vi "Main.vi"() -> ()   [LabVIEW 2015]
uses:
  Game States.ctl
  Game Data.ctl
  <vilib>/MakerHub/LINX/Private/Type Defs/User Platform.ctl
  <vilib>/MakerHub/LINX/Private/Type Defs/Interface.ctl
  <vilib>/Utility/miscctls.llb/LV3DPointTypeDef.ctl
  3D Point.ctl
  Level/Level.lvclass/Level.ctl
  <vilib>/MakerHub/LINX/Public/Peripherals/Analog/Analog Read 1 Chan.vi
  Player/Player.lvclass
  Level/Level.lvclass
  3D Object/3D Object.lvclass
  Input/Input.lvclass
  3D Scene/3D Scene.lvclass
  Render Window/Render Window.lvclass
  Control Window/Control Window.lvclass
  <vilib>/MakerHub/LINX/LMH-LINX.lvlib
panel:
  out "Step?":bool
  in  "Use Hardware":bool
  out "Error Out":errorcluster
  in  "Error In":errorcluster
  in  "Serial Port":refnum<visa-resource-name>="COM4"
  out "Yaw":sgl
  out "Pitch":sgl
  out "error out":errorcluster
  in  "Display":enum16{"Control Window", "Render Window"}(ring)
  out "3D Debug":refnum<vi>(3d-picture)
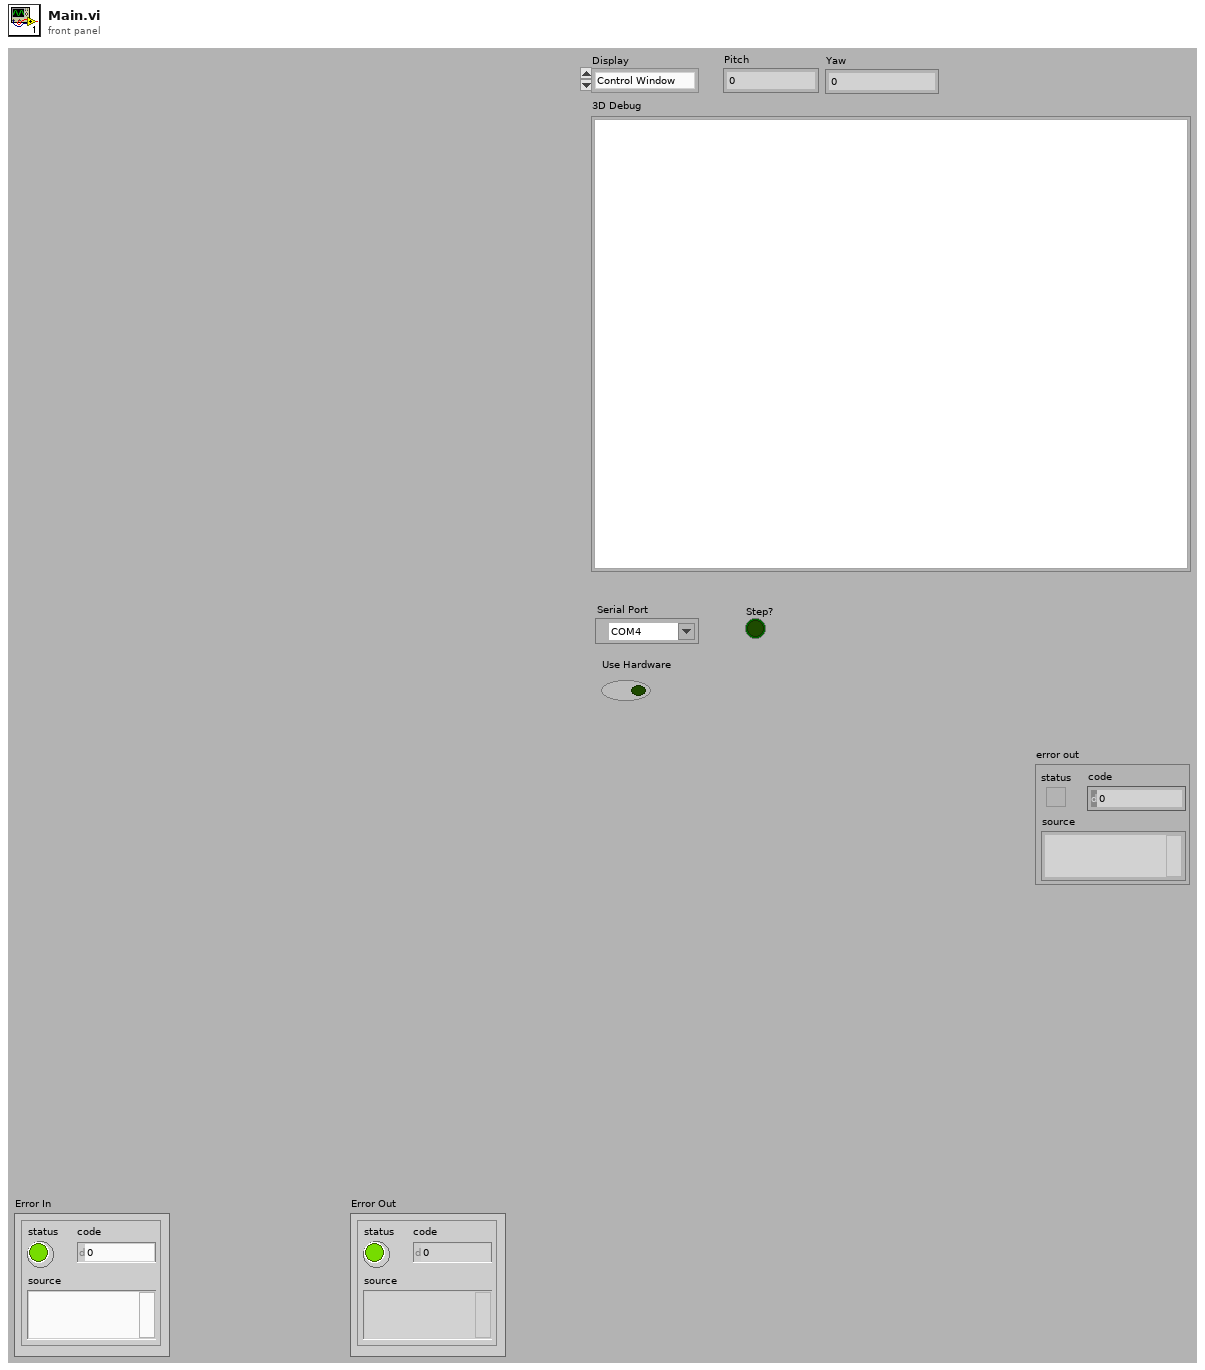
[diagram p1: front panel]
types:
  T1 = typedef "Game Data.ctl" = cluster{"Current Tick Count":u32, "Ticks From Start":u32}
  T2 = typedef "Game States.ctl" = enum16{"Initialize", "Get Input", "Draw Scene", "Shutdown"}
  T3 = typedef "LMH-LINX.lvlib/Interface.ctl" = enum16{"Serial", "TCP"}
  T4 = typedef "LMH-LINX.lvlib/User Platform.ctl" = enum16{"Default", "LINX", "myRIO"}
  T5 = typedef "LMH-LINX.lvlib/LINX Ref.ctl" = cluster{"Platform":T6, "Interface":T3, "LINX Device Config":T7}
  T6 = typedef "LMH-LINX.lvlib/Platform.ctl" = enum16{"LINX", "myRIO"}
  T7 = typedef "LMH-LINX.lvlib/Device.lvlib/LINX Device Config.ctl" = cluster{"Interface":T3, "COM Port":refnum<visa-resource-name>, "TCP Configuration":T8, "Device Family":u8, "Device ID":u8, "Device Name":string, "TCP Ref":refnum<k5>, "Channels":T9}
  T8 = typedef "LMH-LINX.lvlib/Device.lvlib/TCP Config.ctl" = cluster{"IP Address":string, "Port":u16}
  T9 = typedef "LMH-LINX.lvlib/Channels.ctl" = cluster{"DI":u8[], "DO":u8[], "AI":u8[], "AO":u8[], "PWM":u8[], "QE":u8[], "UART":u8[], "I2C 2":u8[], "SPI":u8[], "CAN":u8[], "Servo":u8[], "AI Ref (V)":dbl, "AO Ref (V)":dbl, "AO Resolution (Bits)":u8}
  T10 = typedef "3D Point.ctl" = cluster{"X":sgl, "Y":sgl, "Z":sgl}
  T11 = typedef "LV3DPointTypeDef.ctl" = cluster{"X":sgl, "Y":sgl, "Z":sgl}
  T12 = enum16{"None", "Spherical", "Flying", "Oriented"}
  T13 = enum16{"Open", "Minimized", "Maximized", "Hidden"}
  T14 = typedef "Level.lvclass/Segment.ctl" = cluster{"Point 1":T15, "Point 2":T15}
  T15 = typedef "Level.lvclass/Point.ctl" = cluster{"Z":dbl, "X":dbl}
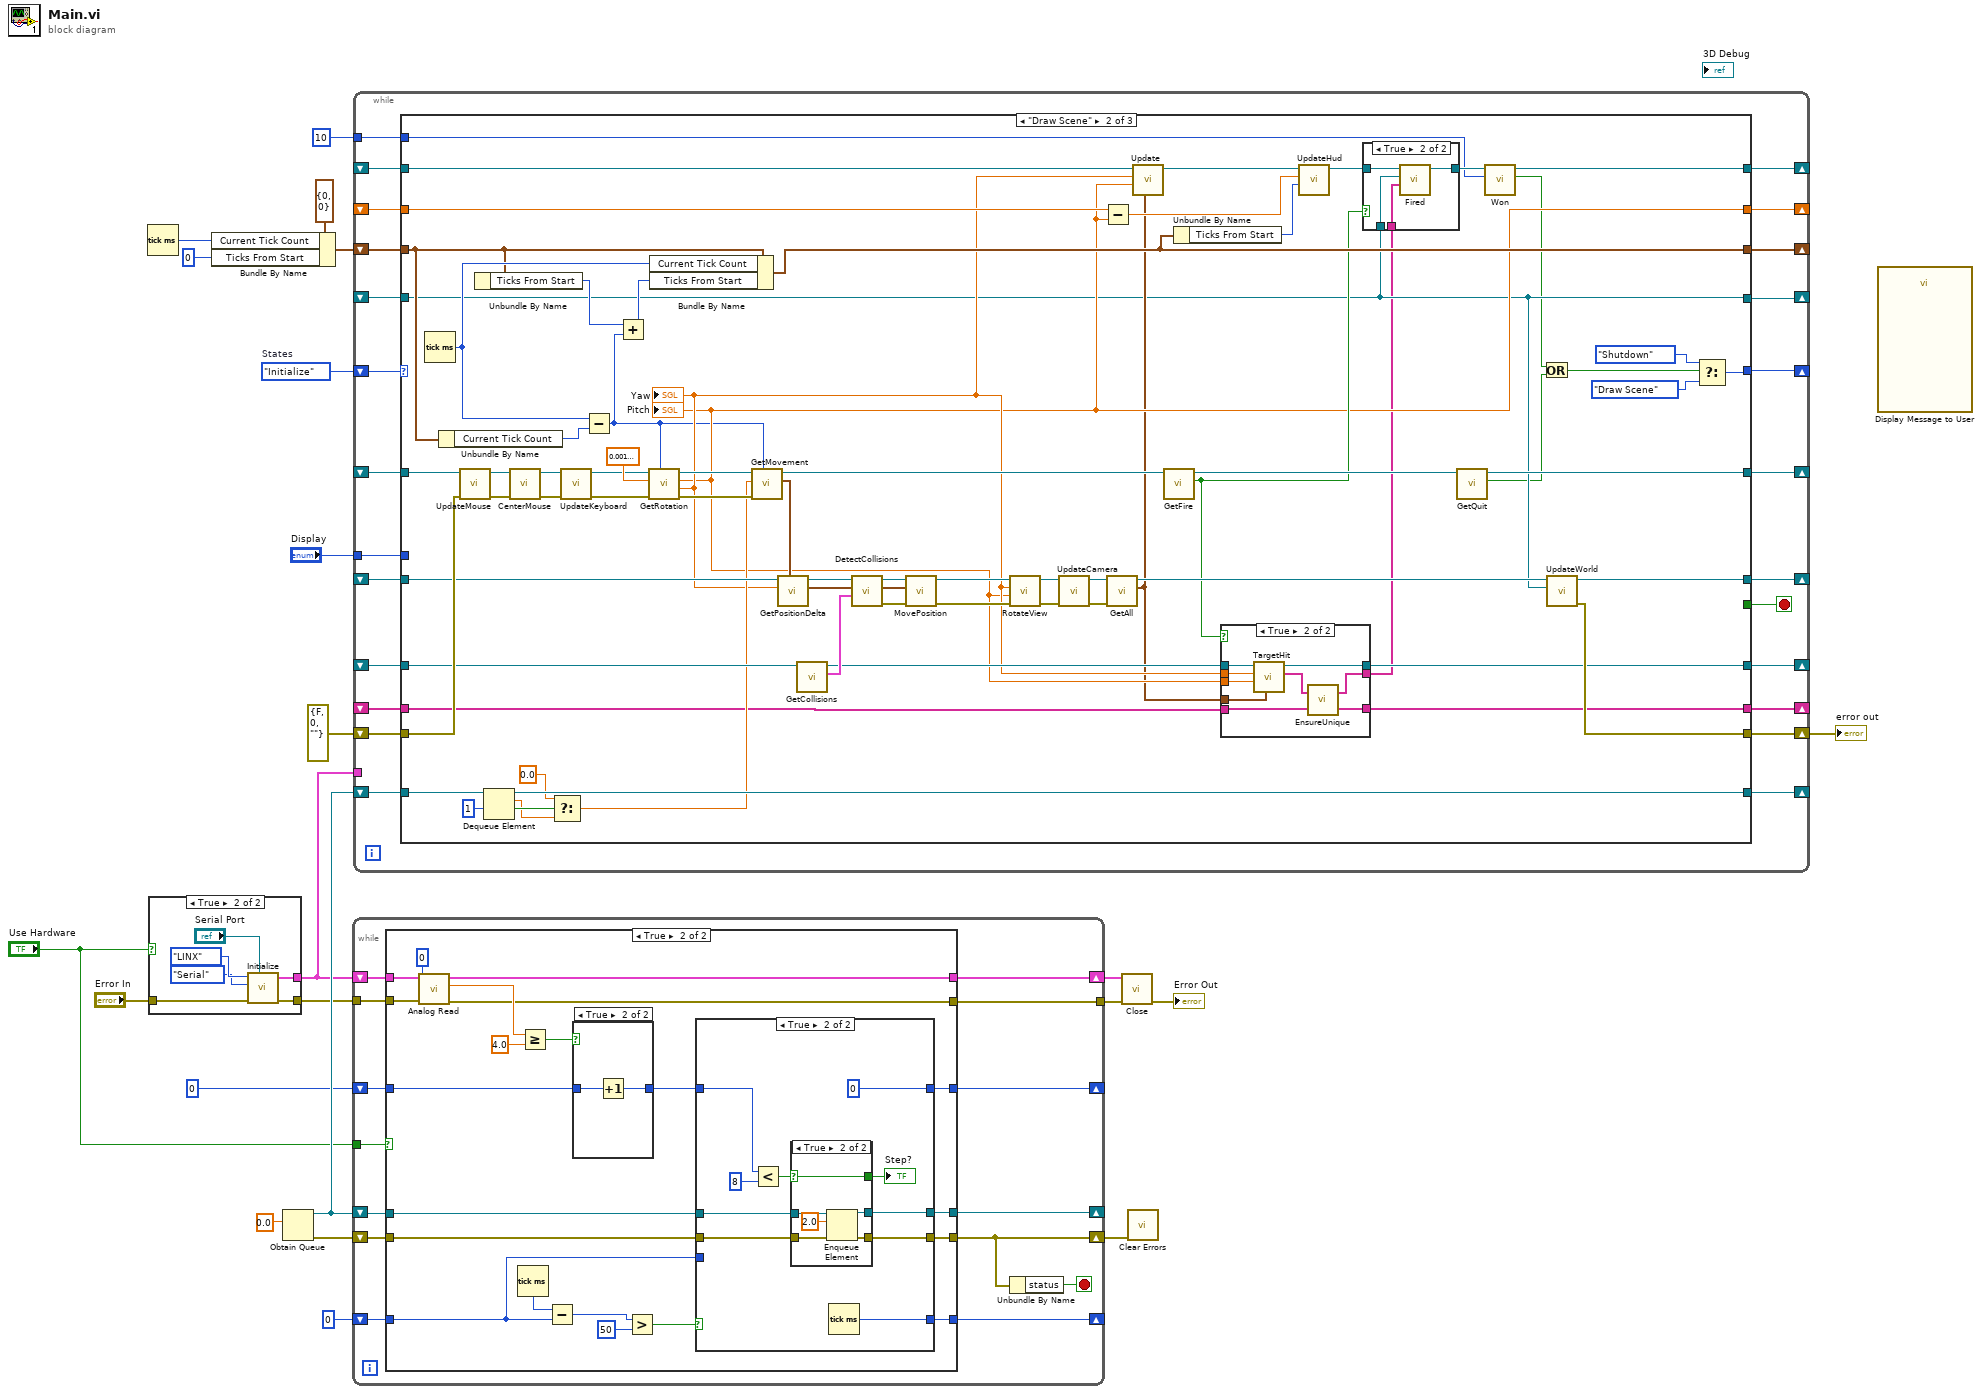
[diagram p0: block diagram]
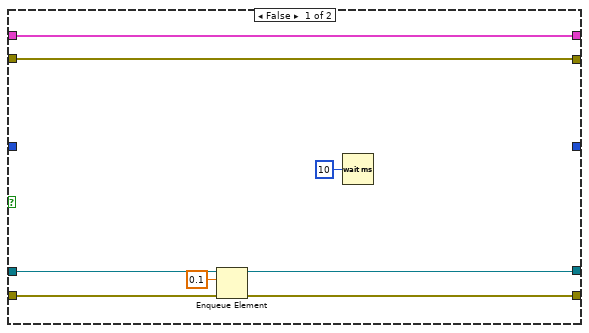
[diagram p3: hidden frame]
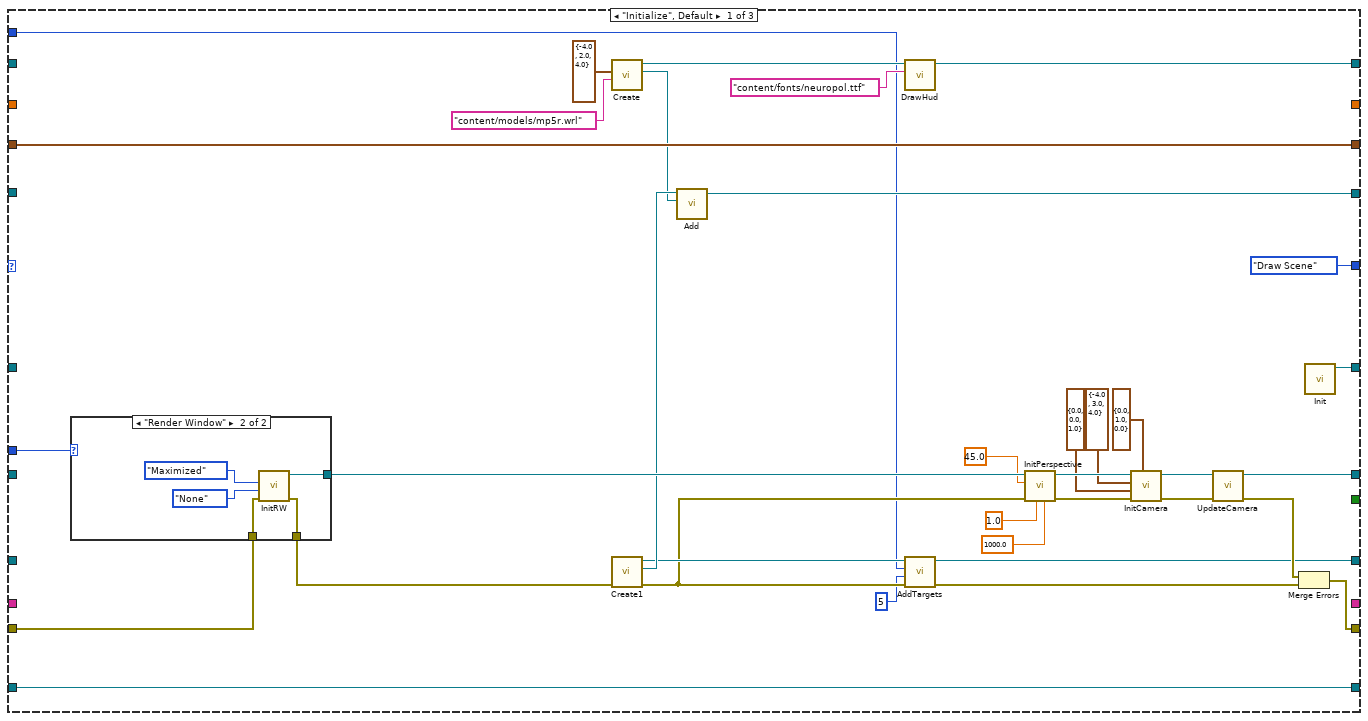
[diagram p7: hidden frame]
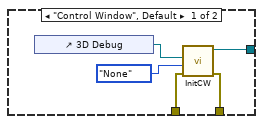
[diagram p8: hidden frame]
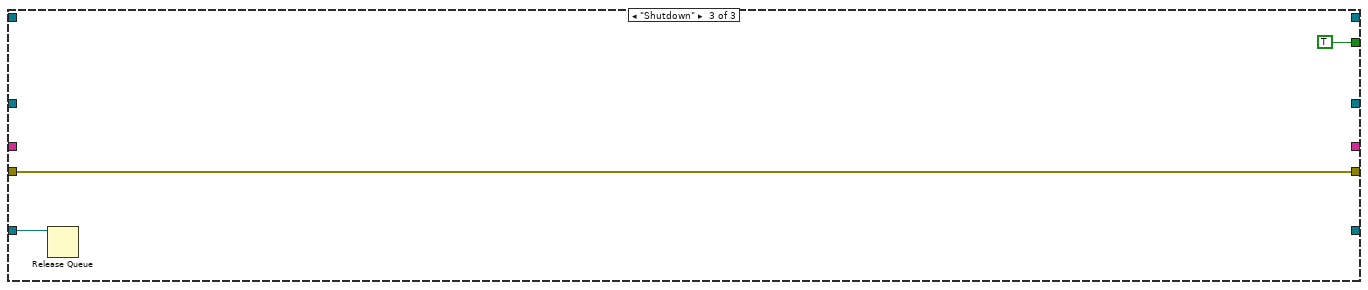
[diagram p11: hidden frame]
diagram:
  w22 = Game_States."Initialize"  # States
  n1 = Tick Count (ms)() -> (millisecond timer value=w3:u32)
  n2 = case shown="True" "Use Hardware" {
    tunnel: [_ w29] -> w15
    tunnel: [w23 w26] -> w11
    tunnel: "Error In" -> [w23 w24]
    frame False {
    }
    frame True {
      n3 = call <vilib>:"Initialize.vi"("Serial Port"="Serial Port", "Error In"=w24, "Interface"=Interface."Serial", "Platform"=User_Platform."LINX") -> ("Error Out"=w26:errorcluster, "LINX Ref"=w29:T5)  [unwired: 5 in, 1 out]
    }
  }
  n4 = Bundle By Name(cluster=T1 {"Current Tick Count"=0, "Ticks From Start"=0} ("Data"), "Current Tick Count"=w3, "Ticks From Start"=u32 0) -> (w18:T1)
  n5 = Obtain Queue(element data type=0.0) -> (queue out=w16:refnum<queue>, error out=w8:errorcluster)  [unwired: 4 in, 1 out]
  n6 = while {
    shift-right: [w42] -> w14
    shift-left: w15 -> [w43]
    shift-right: [w40] -> _
    shift-left: 0 -> [w41]
    shift-right: [w38] -> _
    shift-left: 0 -> [w39]
    tunnel: w11 -> [w37]
    tunnel: [w36] -> w10
    shift-right: [w32] -> w7
    shift-left: w8 -> [w33]
    shift-right: [w34] -> _
    shift-left: w16 -> [w35]
    tunnel: "Use Hardware" -> [w30]
    stop <- w31 stop-if-true
    n7 = case shown="True" w30 {
      tunnel: w43 -> [w51 w72]
      tunnel: [w51 w71] -> w42
      tunnel: w41 -> [_ w66]
      tunnel: [_ w60] -> w40
      tunnel: w39 -> [_ w59]
      tunnel: [_ w58] -> w38
      tunnel: w37 -> [w50 w57]
      tunnel: [w50 w56] -> w36
      tunnel: w35 -> [w49 w55]
      tunnel: [w48 w54] -> w34
      tunnel: w33 -> [w47 w53]
      tunnel: [w46 w52] -> w32
      frame False {
        n8 = Enqueue Element(queue=w49, element=0.1, error in (no error)=w47) -> (queue out=w48:refnum<queue>, error out=w46:errorcluster)  [unwired: 1 in, 1 out]
        n9 = Wait (ms)(milliseconds to wait=u32 10) -> ()  [unwired: 1 out]
      }
      frame True {
        n10 = call-poly <vilib>:"Analog Read.vi"("Error In"=w57, "Analog Channel"=u8 0, "LINX Resource"=w72) -> ("Error Out"=w56:errorcluster, "AI Value"=w69:dbl, "LINX Resource"=w71:T5)  [unwired: 5 in, 1 out]
        n11 = Tick Count (ms)() -> (millisecond timer value=w65:u32)
        n12 = Greater Or Equal?(x=w69, y=4.0) -> (x >= y?=w67:bool)
        n13 = Subtract(x=w65, y=w59) -> (x-y=w64:u32)
        n14 = case shown="True" w67 {
          tunnel: w66 -> [w95 w97]
          tunnel: [w95 w96] -> w61
          frame False {
          }
          frame True {
            n15 = Increment(x=w97) -> (x+1=w96:i32)
          }
        }
        n16 = Greater?(x=w64, y=u32 50) -> (0:w62:bool)
        n17 = case shown="True" w62 {
          tunnel: w61 -> [w76 w84]
          tunnel: [w76 0] -> w60
          tunnel: w59 -> [w75 _]
          tunnel: [w75 w85] -> w58
          tunnel: w55 -> [w74 w82]
          tunnel: [w74 w81] -> w54
          tunnel: w53 -> [w73 w80]
          tunnel: [w73 w79] -> w52
          frame False {
          }
          frame True {
            n18 = Less?(x=w84, y=8) -> (x < y?=w78:bool)
            n19 = case shown="True" w78 {
              selector: w78 -> [_ w89]
              tunnel: w82 -> [w88 w94]
              tunnel: [w88 w93] -> w81
              tunnel: w80 -> [w87 w92]
              tunnel: [w87 w91] -> w79
              tunnel: [_ w89] -> w77
              frame False {
              }
              frame True {
                n20 = Enqueue Element(queue=w94, element=2.0, error in (no error)=w92) -> (queue out=w93:refnum<queue>, error out=w91:errorcluster)  [unwired: 1 in, 1 out]
              }
            }
            "Step?" <- w77
            n21 = Tick Count (ms)() -> (millisecond timer value=w85:u32)
          }
        }
      }
    }
    n22 = Unbundle By Name(w32) -> ("status"=w31:bool)
  }
  n23 = while {
    shift-right: [w121] -> _
    shift-left: w22 -> [w122]
    tunnel: "Display" -> [w119]
    shift-right: [w118] -> _
    shift-left: _ -> [w117]
    shift-right: [w115] -> _
    shift-left: _ -> [w114]
    shift-right: [w112] -> _
    shift-left: w18 -> [w113]
    shift-right: [w111] -> _
    shift-left: _ -> [w110]
    shift-right: [w107] -> _
    shift-left: _ -> [w108]
    shift-right: [w109] -> w17
    shift-left: errorcluster {"status"=FALSE, "code"=0, "source"=""} ("error in (no error)") -> [w116]
    shift-right: [w105] -> _
    shift-left: w16 -> [w106]
    tunnel: w15 -> [_]
    shift-right: [w104] -> _
    shift-left: _ -> [w103]
    shift-right: [w102] -> _
    shift-left: _ -> [w101]
    tunnel: 10 ("Num Targets") -> [w100]
    shift-right: [w98] -> _
    shift-left: _ -> [w99]
    stop <- w120 stop-if-true
    n24 = case shown="\"Draw Scene\"" w122 {
      tunnel: [Game_States."Draw Scene" ("States") w232 _] -> w121
      tunnel: [_ _ TRUE] -> w120
      tunnel: w119 -> [w156 _ _]
      tunnel: [w147 w230 _] -> w118
      tunnel: w117 -> [_ w205 _]
      tunnel: w116 -> [w140 w218 w256]
      tunnel: [w149 w234 _] -> w115
      tunnel: w114 -> [_ w229 _]
      tunnel: w113 -> [w152 w191 _]
      tunnel: [w152 w192 _] -> w112
      tunnel: [w145 w178 _] -> w111
      tunnel: w110 -> [_ w178 _]
      tunnel: [w136 w227 w256] -> w109
      tunnel: w108 -> [_ w209 _]
      tunnel: [w125 w183 _] -> w107
      tunnel: w106 -> [w141 w204 w255]
      tunnel: [w141 w202 _] -> w105
      tunnel: [w130 w176 _] -> w104
      tunnel: w103 -> [_ w197 _]
      tunnel: [_ w180 _] -> w102
      tunnel: w101 -> [_ w195 _]
      tunnel: w100 -> [w123 w175 _]
      tunnel: w99 -> [_ w170 _]
      tunnel: [_ w169 _] -> w98
      frame "Initialize", Default {
        n25 = case shown="\"Render Window\"" w156 {
          tunnel: [w160 w165] -> w155
          tunnel: w140 -> [w159 w164]
          tunnel: [w158 w163] -> w139
          frame "Control Window", Default {
            n26 = control-ref of="3D Debug"() -> (w161:refnum<vi>)
            n27 = call "InitCW.vi"("error in (no error)"=w159, "Camera Controller"=T12."None", "SceneGraphDisp"=w161) -> ("error out"=w158:errorcluster, "Control Window out"=w160:refnum<class "Control Window.lvclass">)  [unwired: 7 in]
          }
          frame "Render Window" {
            n28 = call "InitRW.vi"("error in (no error)"=w164, "Camera Controller"=enum16{"None", "Spherical", "Flying"}."None", "Window State"=T13."Maximized") -> ("error out"=w163:errorcluster, "Render Window out"=w165:refnum<class "Render Window.lvclass">)  [unwired: 7 in]
          }
        }
        n29 = call "Create.vi"("Gun VRML"="content/models/mp5r.wrl", "Position"=T10 {"X"=-4.0, "Y"=2.0, "Z"=4.0}) -> ("Model"=w132:refnum<class "3D Object.lvclass">, "Player out"=w131:refnum<class "Player.lvclass">)  [unwired: 7 in, 1 out]
        n30 = call "Create1.vi"("error in (no error)"=w139) -> ("error out"=w127:errorcluster, "Model"=w133:refnum<class "3D Object.lvclass">, "Level out"=w128:refnum<class "Level.lvclass">)  [unwired: 8 in]
        n31 = call "Add.vi"("Child in"=w132, "Parent in"=w133) -> ("Parent out"=w145:refnum<class "3D Object.lvclass">)  [unwired: 7 in, 2 out]
        n32 = call "DrawHud.vi"("Font"="content/fonts/neuropol.ttf", "Player in"=w131) -> ("Player out"=w130:refnum<class "Player.lvclass">)  [unwired: 8 in, 1 out]
        n33 = call "AddTargets.vi"("error in (no error)"=w127, "Difficulty"=u8 5, "Num Targets"=w123, "Level in"=w128) -> ("error out"=w126:errorcluster, "Level out"=w125:refnum<class "Level.lvclass">)  [unwired: 6 in]
        n34 = call-dynamic "InitPerspective.vi"("Far Clipping"=sgl 1000.0, "Near Clipping"=sgl 1.0, "error in (no error)"=w127, "FOV"=sgl 45.0, "3D Scene in"=w155) -> ("error out"=w143:errorcluster, "3D Scene out"=w151:refnum<class "3D Scene.lvclass">)  [unwired: 5 in]
        n35 = call "InitCamera.vi"("Up Direction"=T11 {"X"=0.0, "Y"=1.0, "Z"=0.0}, "error in (no error)"=w143, "Target"=T11 {"X"=0.0, "Y"=0.0, "Z"=1.0}, "Camera Position"=T11 {"X"=-4.0, "Y"=3.0, "Z"=4.0}, "3D Scene in"=w151) -> ("error out"=w144:errorcluster, "3D Scene out"=w148:refnum<class "3D Scene.lvclass">)  [unwired: 5 in]
        n36 = call-dynamic "UpdateCamera.vi"("error in (no error)"=w144, "3D Scene in"=w148) -> ("error out"=w137:errorcluster, "3D Scene out"=w147:refnum<class "3D Scene.lvclass">)  [unwired: 8 in]
        n37 = Merge Errors(w137, w126) -> (w136:errorcluster)
        n38 = call "Init.vi"() -> ("Input out"=w149:refnum<class "Input.lvclass">)  [unwired: 10 in, 1 out]
      }
      frame "Draw Scene" {
        n39 = Tick Count (ms)() -> (millisecond timer value=w235:u32)
        n40 = Unbundle By Name(w191) -> ("Current Tick Count"=w236:u32)
        n41 = call "UpdateMouse.vi"("error in (no error)"=w218, "Input in"=w229) -> ("error out"=w225:errorcluster, "Input out"=w226:refnum<class "Input.lvclass">)  [unwired: 8 in]
        n42 = Unbundle By Name(w191) -> ("Ticks From Start"=w190:u32)
        n43 = Dequeue Element(queue=w204, timeout in ms (-1)=1) -> (queue out=w202:refnum<queue>, element=w200:dbl, timed out?=w201:bool)  [unwired: 1 in, 1 out]
        n44 = call "CenterMouse.vi"("error in (no error)"=w225, "Input in"=w226) -> ("error out"=w221:errorcluster, "Input out"=w224:refnum<class "Input.lvclass">)  [unwired: 8 in]
        n45 = Select(t=0.0, s=w201, f=w200) -> (s? t:f=w199:dbl)
        n46 = call "UpdateKeyboard.vi"("error in (no error)"=w221, "Input in"=w224) -> ("error out"=w222:errorcluster, "Input out"=w223:refnum<class "Input.lvclass">)  [unwired: 8 in]
        n47 = Subtract(x=w235, y=w236) -> (x-y=w168:u32)
        n48 = Add(x=w190, y=w168) -> (x+y=w189:u32)
        n49 = call "GetRotation.vi"("Game Ticks"=w168, "error in (no error)"=w222, "Rotation Speed"=sgl 0.001, "Input in"=w223) -> ("error out"=w228:errorcluster, "Yaw"=w181:sgl, "Pitch"=w180:sgl, "Input out"=w237:refnum<class "Input.lvclass">)  [unwired: 4 in]
        "Pitch" <- w180
        "Yaw" <- w181
        n50 = Bundle By Name(cluster=w191, "Current Tick Count"=w235, "Ticks From Start"=w189) -> (w192:T1)
        n51 = call "GetMovement.vi"("Game Ticks"=w168, "error in (no error)"=w228, "Move Speed"=w199, "Input in"=w237) -> ("Move Vector"=w213:cluster{"[0]":sgl, "[1]":sgl, "[2]":sgl}, "Input out"=w188:refnum<class "Input.lvclass">)  [unwired: 5 in, 1 out]
        n52 = call "GetPositionDelta.vi"("Move Vector"=w213, "Yaw"=w181, "3D Scene in"=w205) -> ("Position Delta"=w207:cluster{"X":sgl, "Y":sgl, "Z":sgl}, "3D Scene out"=w212:refnum<class "3D Scene.lvclass">)  [unwired: 6 in, 1 out]
        n53 = call "GetCollisions.vi"("Level in"=w209) -> ("Collisions"=w208:T14[], "Level out"=w184:refnum<class "Level.lvclass">)  [unwired: 8 in, 1 out]
        n54 = call "DetectCollisions.vi"("Collision Points"=w208, "Position Delta"=w207, "3D Scene in"=w212) -> ("error out"=w210:errorcluster, "Adjusted Position Delta"=w206:cluster{"X":sgl, "Y":sgl, "Z":sgl}, "3D Scene out"=w211:refnum<class "3D Scene.lvclass">)  [unwired: 6 in]
        n55 = call "MovePosition.vi"("error in (no error)"=w210, "Position Delta"=w206, "3D Scene in"=w211) -> ("error out"=w216:errorcluster, "3D Scene out"=w217:refnum<class "3D Scene.lvclass">)  [unwired: 7 in]
        n56 = call "RotateView.vi"("error in (no error)"=w216, "Pitch"=w180, "Yaw"=w181, "3D Scene in"=w217) -> ("error out"=w214:errorcluster, "3D Scene out"=w215:refnum<class "3D Scene.lvclass">)  [unwired: 6 in]
        n57 = call-dynamic "UpdateCamera.vi"("error in (no error)"=w214, "3D Scene in"=w215) -> ("error out"=w219:errorcluster, "3D Scene out"=w220:refnum<class "3D Scene.lvclass">)  [unwired: 8 in]
        n58 = Subtract(x=w195, y=w180) -> (x-y=w194:sgl)
        n59 = call "GetAll.vi"("error in (no error)"=w219, "3D Scene in"=w220) -> ("Position"=w179:T10, "3D Scene out"=w185:refnum<class "3D Scene.lvclass">)  [unwired: 5 in, 3 out]
        n60 = call "Update.vi"("New Position"=w179, "Pitch"=w180, "Yaw"=w181, "Player in"=w197) -> ("Player out"=w196:refnum<class "Player.lvclass">)  [unwired: 6 in, 1 out]
        n61 = call "GetFire.vi"("Input in"=w188) -> ("Fire?"=w182:bool, "Input out"=w187:refnum<class "Input.lvclass">)  [unwired: 8 in, 1 out]
        n62 = Unbundle By Name(w192) -> ("Ticks From Start"=w193:u32)
        n63 = case shown="True" w182 {
          tunnel: w184 -> [w240 w249]
          tunnel: [w240 w248] -> w183
          tunnel: w181 -> [_ w247]
          tunnel: w180 -> [_ w246]
          tunnel: w179 -> [_ w245]
          tunnel: [_ w243] -> w171
          tunnel: w170 -> [w239 w241]
          tunnel: [w239 w242] -> w169
          frame False {
          }
          frame True {
            n64 = call "TargetHit.vi"("Position"=w245, "Pitch"=w246, "Yaw"=w247, "Level in"=w249) -> ("Hit Targets"=w244:string[], "Level out"=w248:refnum<class "Level.lvclass">)  [unwired: 5 in, 1 out]
            n65 = call "EnsureUnique.vi"("Existing Targets Hit"=w241, "Potentially New Targets Hit"=w244) -> ("Existing Targets Hit Updated"=w242:string[], "New Targets Hit"=w243:string[])
          }
        }
        n66 = call "UpdateHud.vi"("Ticks Elapsed (ms)"=w193, "Pitch Delta"=w194, "Player in"=w196) -> ("Player out"=w186:refnum<class "Player.lvclass">)  [unwired: 7 in, 1 out]
        n67 = case shown="True" w182 {
          tunnel: w186 -> [w250 w254]
          tunnel: [w250 w253] -> w177
          tunnel: w171 -> [_ w252]
          tunnel: w178 -> [_ w251]
          frame False {
          }
          frame True {
            n68 = call "Fired.vi"("Hit Targets"=w252, "World In"=w251, "Player in"=w254) -> ("Player out"=w253:refnum<class "Player.lvclass">)  [unwired: 7 in, 1 out]
          }
        }
        n69 = call "GetQuit.vi"("Input in"=w187) -> ("Quit?"=w174:bool, "Input out"=w234:refnum<class "Input.lvclass">)  [unwired: 8 in, 1 out]
        n70 = call "Won.vi"("Num Targets"=w175, "Player in"=w177) -> ("Won?"=w173:bool, "Player out"=w176:refnum<class "Player.lvclass">)  [unwired: 7 in, 1 out]
        n71 = Or(x=w173, y=w174) -> (x .or. y?=w172:bool)
        n72 = call-dynamic "UpdateWorld.vi"("World in"=w178, "3D Scene in"=w185) -> ("error out"=w227:errorcluster, "3D Scene out"=w230:refnum<class "3D Scene.lvclass">)  [unwired: 8 in]
        n73 = Select(t=Game_States."Shutdown" ("States"), s=w172, f=Game_States."Draw Scene") -> (s? t:f=w232:T2)
      }
      frame "Shutdown" {
        n74 = Release Queue(queue=w255) -> ()  [unwired: 2 in, 3 out]
      }
    }
  }
  "error out" <- w17
  n75 = call <vilib>:"Close.vi"("Error In"=w10, "LINX Resource"=w14) -> ("Error Out"=→"Error Out":errorcluster)  [unwired: 8 in, 1 out]
  n76 = call <vilib>:"Clear Errors.vi"("error in (no error)"=w7) -> ()  [unwired: 5 in, 2 out]
  n77 = call "Display Message to User"() -> ()  [unwired: 10 in, 2 out]
